vi "Set queue.vi"(8 "error in (no error)":errorcluster {"code" format="Error %.0f"}, 10 "queue":string, 11 "NATS Subscription in":refnum<class "NATS Subscription.lvclass">) -> (0 "error out":errorcluster {"code" format="Error %.0f"}, 3 "NATS Subscription out":refnum<class "NATS Subscription.lvclass">)   [LabVIEW 2020, in "NATS Subscription.lvlib" / "NATS Subscription.lvclass"]
uses:
  NATS Subscription.lvclass
  NATS Subscription.lvclass/NATS Subscription.ctl
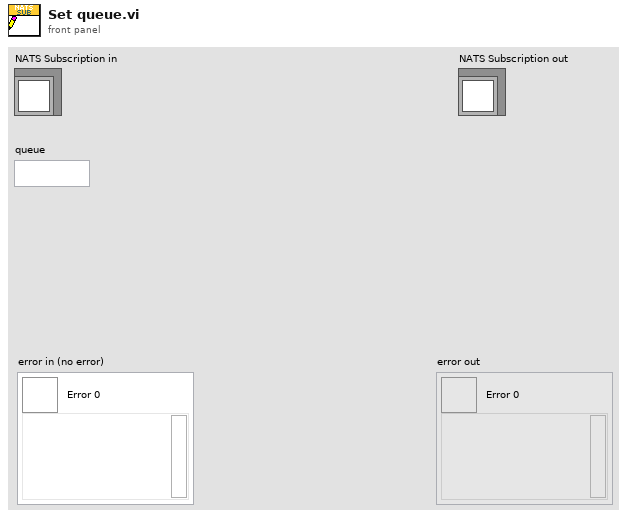
[diagram p1: front panel]
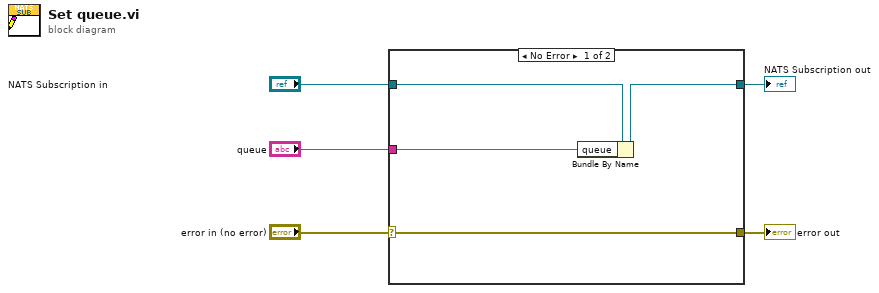
[diagram p0: block diagram]
diagram:
  n1 = case shown="No Error" "error in (no error)" {
    selector: "error in (no error)" -> [w9 w10]
    tunnel: [w9 w10] -> w4
    tunnel: [w7 w11] -> w2
    tunnel: "NATS Subscription in" -> [w8 w11]
    tunnel: "queue" -> [w6 _]
    frame No Error {
      n2 = Bundle By Name(cluster=w8, "queue"=w6) -> (w7:refnum<class "NATS Subscription.lvclass">)
    }
    frame Error {
    }
  }
  "error out" <- w4
  "NATS Subscription out" <- w2
